vi "GetControlReference.vi"(8 "error in":errorcluster, 11 "Control in":refnum<class "Control.lvclass">) -> (0 "error out":errorcluster, 1 "control reference":refnum<vi>, 3 "Control out":refnum<class "Control.lvclass">)   [LabVIEW 2014, in "Control.lvclass"]
uses:
  Control.lvclass
  Generic/Generic.lvclass
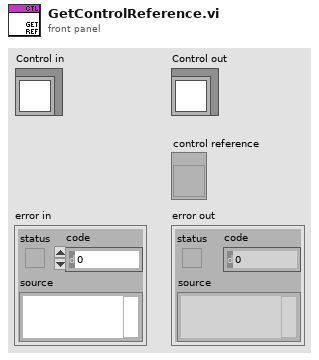
[diagram p1: front panel]
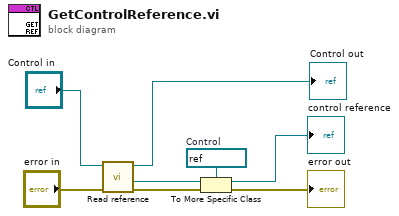
[diagram p0: block diagram]
diagram:
  w8 = refnum<vi> refnum  # Control
  n1 = call "Read reference.vi"("error in"="error in", "GObject in"="Control in") -> ("error out"=w3:errorcluster, "reference"=w2:refnum<vi>, "GObject out"=→"Control out":refnum<class "Control.lvclass">)  [unwired: 5 in]
  n2 = To More Specific Class(target class=w8, reference=w2, error in=w3) -> (specific class reference=→"control reference":refnum<vi>, error out=→"error out":errorcluster)
